vi "运维调试_氨氮.vi"() -> ()   [LabVIEW 2016, in "斯坦道氨氮.lvlib"]
uses:
  <vilib>/Utility/miscctls.llb/LVPointTypeDef.ctl
  <vilib>/Utility/config.llb/NI_LVConfig.lvlib
  <vilib>/ptbypt/NI_PtbyPt.lvlib
panel:
  out "二级权限":bool
  out "一级权限":bool
  out "输入密码":u32
  out "布尔":bool
  in  "仪器参数设置":bool
  in  "流程固件":bool
  in  "量程参数读取":T1
  in  "模块启用":bool
  in  "串口设置":bool
  in  "公式一键写入":bool
  in  "流程路径":path=path "C:/Users/STD/Documents/斯坦道流程文件/流程.xml"
  in  "曲线模型":cluster{"X^2":dbl, "X":dbl, "B":dbl}(xcontrol)
  out "字符串":string
  in  "质控参数设置":bool
  in  "自动测试量程配置":T2
  out "温度2":sgl
  out "温度1":sgl
  out "ADC":sgl
  out "固件版本号":string
  in  "数组":string[](array[string])
  in  "量程切换阈值写入":bool
  in  "量程切换阈值读取":bool
  in  "参数下拉列表":enum16{"总磷", "总氮", "氨氮"}(ring)=enum."氨氮"
  in  "量程下拉列表":enum16{"低量程", "高量程"}(ring)
  in  "测量模式下拉列表":enum16{"水样测量", "零点核查", "跨度核查", "标样核查", "加标回收"}(ring)
  in  "公式":cluster{"X^2":dbl, "X":dbl, "b":dbl}
  in  "写公式":bool
  in  "读公式":bool
  in  "返回":bool
  in  "设置":bool
  out "序列号":string="序列号"
  out "测量数据":T3(xcontrol)
  out "集成报警信息":string
  out "定时启动":bool
  out "总磷总氮运行状态":T4(xcontrol)
  in  "停止":bool
  in  "手动启动":bool
  in  "单步测试":bool
  in  "总磷氨氮调试":u16[](xcontrol)
  out "F3":sgl format="%#.6f"
  out "F2":sgl format="%#.6f"
  out "F1":sgl format="%#.6f"
  out "F0":sgl format="%#.6f"
  out "多列列表框":i32(listbox)
  # "参数设置"
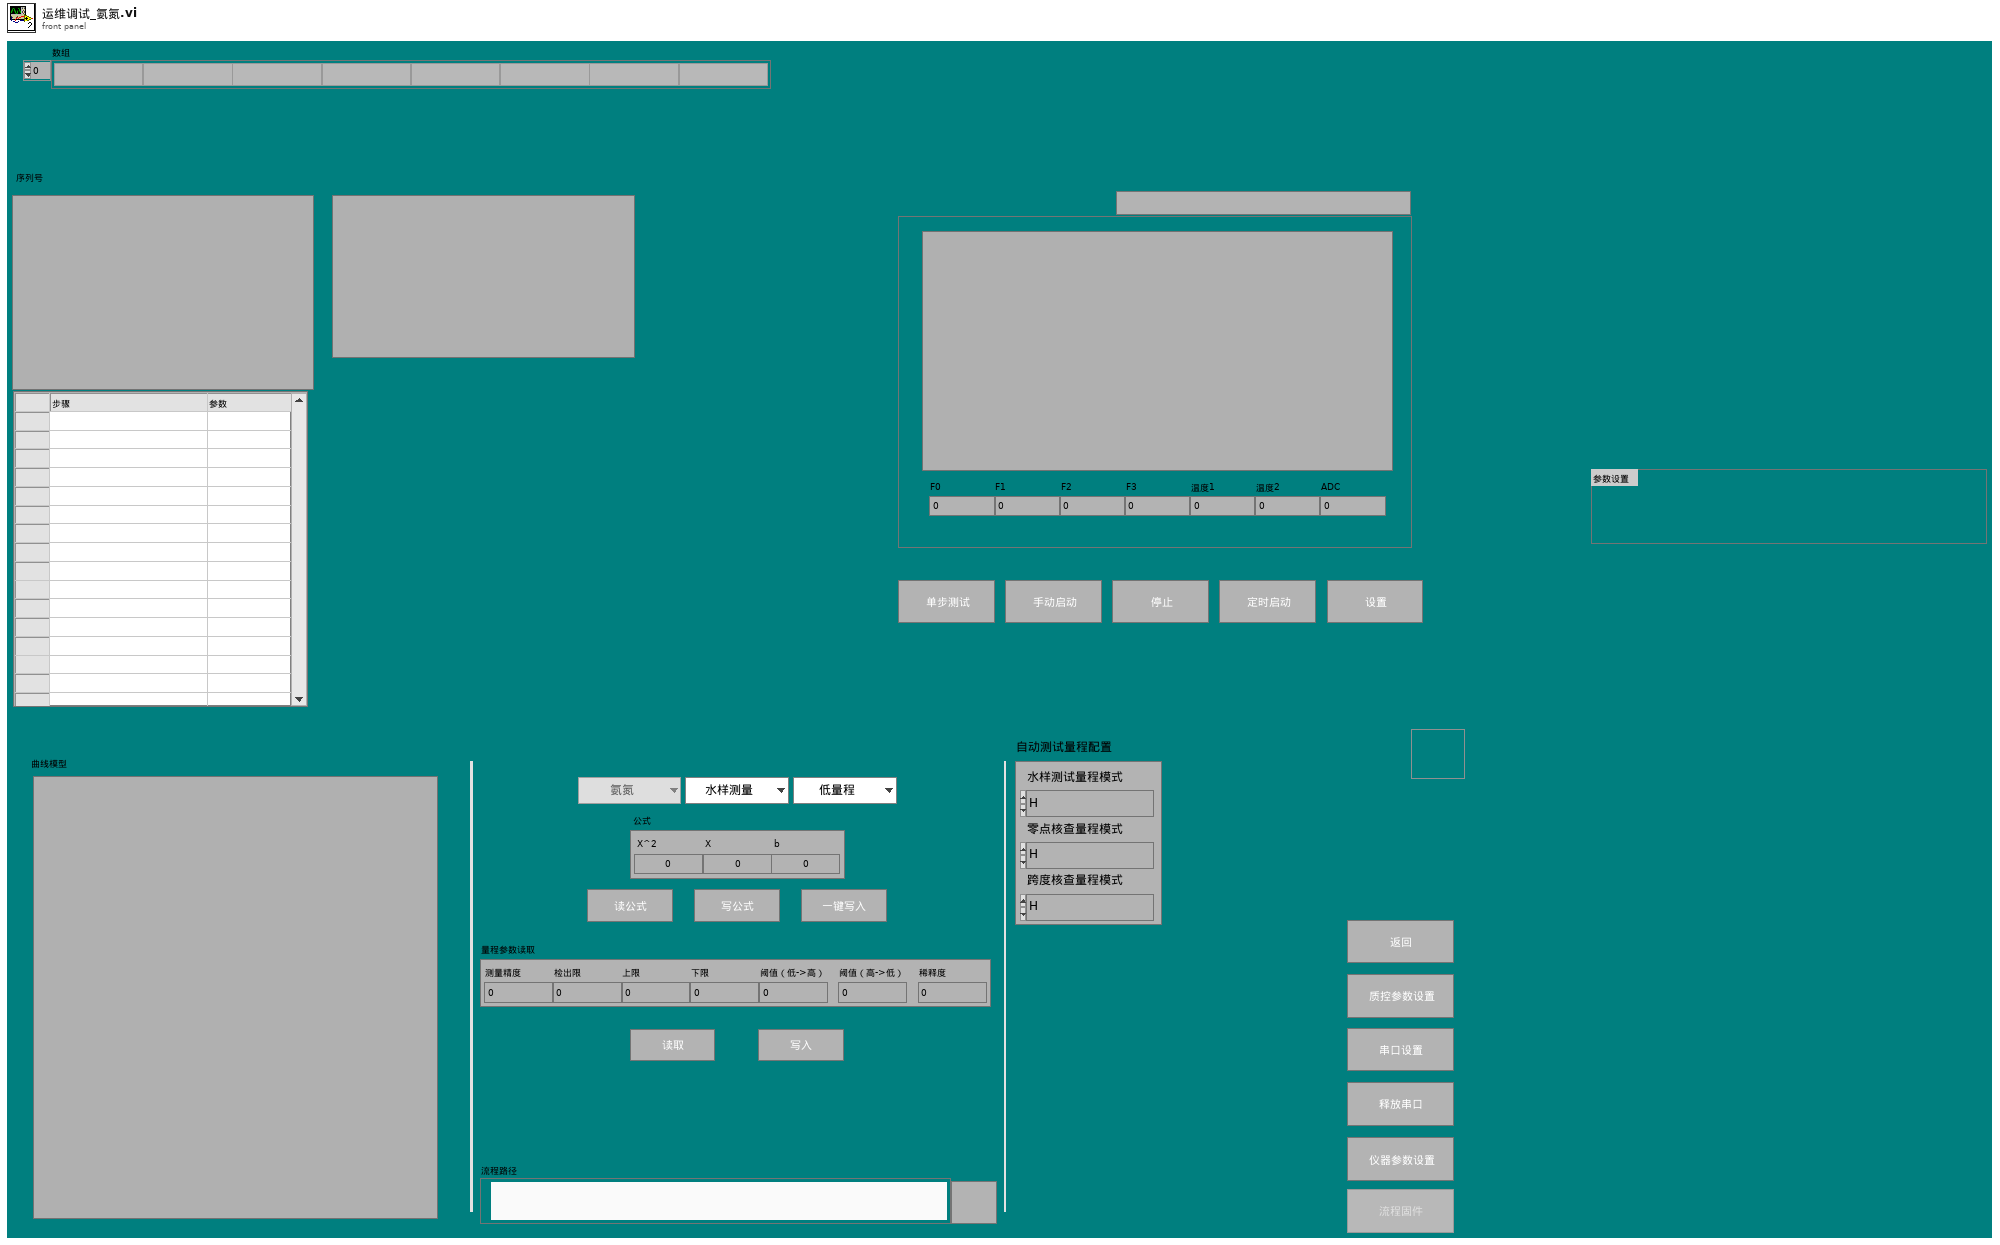
[diagram p1: front panel]
types:
  T1 = cluster{"测量精度":dbl, "检出限":dbl, "上限":dbl, "下限":dbl, "阈值（低->高）":dbl, "阈值（高->低）":dbl, "稀释度":dbl}
  T2 = cluster{"水样测试量程模式":enum16{"H", "L", "AUTO"}, "空白核查量程模式":enum16{"H", "L", "AUTO"}, "跨度核查量程模式":enum16{"H", "L", "AUTO"}}
  T3 = cluster{"flowid":u16, "测量精度":u16, "测量数据区":cluster{"因子编码":u32, "单位":u16, "标样参考值":sgl, "水样数据时间":timestamp, "水样实测值":sgl, "水样数据标识":string, "标样数据时间":timestamp, "标样实测值":sgl, "标样数据标识":string, "空白数据时间":timestamp, "空白实测值":sgl, "空白数据标识":string, "零点核查数据时间":timestamp, "零点核查实测值":sgl, "零点核查数据标识":string, "跨度核查数据时间":timestamp, "跨度核查实测值":sgl, "跨度核查数据标识":string, "加标回收数据时间":timestamp, "加标回收实测值":sgl, "加标回收数据标识":string, "平行样数据时间":timestamp, "平行样实测值":sgl, "平行样数据标识":string, "F0":sgl, "F1":sgl, "F2":sgl, "F3":sgl, "F4":sgl, "F5":sgl, "F6":sgl, "F7":sgl, "温度":sgl, "湿度":sgl, "X值":sgl, "fidrange":sgl}}
  T4 = cluster{"系统时间":timestamp, "工作状态":enum16{"空闲", "水样测试", "标样核查", "零点核查", "跨度核查", "空白测试", "平行样测试", "加标回收", "空白校准", "标样校准", "初始化（清洗）"}, "测量模式":enum16{"待机", "连续模式", "周期模式", "定点模式", "受控模式", "手动模式"}, "告警代码":u16, "故障代码":u16, "日志代码":u16, "软件版本":u16, "F0":sgl, "F1":sgl, "F2":sgl, "F3":sgl, "T":sgl, "H":sgl, "id":u16, "flowid":u16, "量程":u16, "总磷控温温度1":sgl, "营养盐控温温度2":sgl, "ADC":sgl}
  T5 = enum16{"启动测量", "标样核查", "零点核查", "跨度核查", "空白测试", "平行样测试", "加标回收", "空白校准", "标样校准", "初始化（清洗）", "停止测试", "仪器重启", "校时", "模式设置", "测量间隔设置"}
  T6 = cluster{"控制命令":enum16{"启动测量", "标样核查", "零点核查", "跨度核查", "空白测试", "平行样测试", "加标回收", "空白校准", "标样校准", "初始化（清洗）", "停止测试", "仪器重启", "校时", "模式设置", "测量间隔设置"}, "周期设置类型":enum16{"定点启动", "间隔启动"}, "定时功能启用":bool, "定时间隔":dbl, "24H周期设置":bool[], "零点核查时间":u16, "跨度核查时间":u16, "质控频次":enum16{"关闭", "每天", "星期一", "星期二", "星期三", "星期四", "星期五", "星期六", "星期日"}}
  T7 = enum16{"关闭", "每天", "星期一", "星期二", "星期三", "星期四", "星期五", "星期六", "星期日"}
  T8 = typedef "LVDateTimeRec.ctl" = cluster{"秒数的小数部分":dbl, "秒":i32, "分":i32, "时":i32, "日":i32, "月":i32, "年":i32, "天数（周）":i32, "天数（年）":i32, "DST":i32}
  T9 = enum16{"空闲", "水样测试", "标样核查", "零点核查", "跨度核查", "空白测试", "平行样测试", "加标回收", "空白校准", "标样校准", "初始化（清洗）"}
  T10 = enum32{"Bad", "Idle", "Run top level", "Running"}
  T11 = typedef "LVPointTypeDef.ctl" = cluster{"Horizontal":i16, "Vertical":i16}
  T12 = cluster{"因子编码":u32, "单位":u16, "标样参考值":sgl, "水样数据时间":timestamp, "水样实测值":sgl, "水样数据标识":string, "标样数据时间":timestamp, "标样实测值":sgl, "标样数据标识":string, "空白数据时间":timestamp, "空白实测值":sgl, "空白数据标识":string, "零点核查数据时间":timestamp, "零点核查实测值":sgl, "零点核查数据标识":string, "跨度核查数据时间":timestamp, "跨度核查实测值":sgl, "跨度核查数据标识":string, "加标回收数据时间":timestamp, "加标回收实测值":sgl, "加标回收数据标识":string, "平行样数据时间":timestamp, "平行样实测值":sgl, "平行样数据标识":string, "F0":sgl, "F1":sgl, "F2":sgl, "F3":sgl, "F4":sgl, "F5":sgl, "F6":sgl, "F7":sgl, "温度":sgl, "湿度":sgl, "X值":sgl, "fidrange":u16}
  T13 = typedef "NI_LVConfig.lvlib/Config Data RefNum.ctl" = refnum<k1>
  T14 = enum8{"Enabled", "Disabled", "Disabled and Grayed Out"}
  T15 = cluster{"启动模式":enum16{"跨度核查", "水样测量", "空白核查", "标样核查", "加标回收"}, "启动参数":u16, "量程":enum16{"低量程", "高量程"}}
  T16 = cluster{"时间标识":timestamp, "设备":string, "日志信息":string, "流程参数":string}
  T17 = cluster{"时间标识":timestamp, "设备":string, "日志信息":string}
  T18 = typedef "LVRowAndColumnUnsignedTypeDef.ctl" = cluster{"Row":u32, "Column":u32}
  T19 = cluster{"参数下拉列表":enum16{"总磷", "总氮", "氨氮"}, "测量模式下拉列表":enum16{"水样测量", "零点核查", "跨度核查", "标样核查", "加标回收"}, "量程下拉列表":enum16{"低量程", "高量程"}}
  T20 = cluster{"站号":u16, "量程切换":enum32{"H", "L", "AUTO"}, "控制命令":enum16{"启动测量", "标样核查", "零点核查", "跨度核查", "空白测试", "平行样测试", "加标回收", "空白校准", "标样校准", "初始化（清洗）", "停止测试", "仪器重启", "校时", "模式设置", "测量间隔设置"}, "模式设置":enum16{"待机", "连续模式", "周期模式", "定点模式", "受控模式", "手动模式"}, "测量间隔":u16}
  T21 = cluster{"跨度值":dbl, "零点标准液浓度":dbl, "跨度标准液浓度":dbl, "标准液标准浓度":dbl}
  T22 = cluster{"确定":bool, "跨度值":dbl, "零点标准液浓度":dbl, "跨度标准液浓度":dbl, "标准液标准浓度":dbl}
  T23 = cluster{"测量量程":dbl, "测量精度":dbl, "测量间隔":dbl, "消解温度":dbl, "消解时长":dbl, "空白校准时间":timestamp, "曲线截距":dbl, "曲线斜率":dbl, "测量检出限":dbl, "测量信号值":dbl, "线性相关系数":dbl, "二次多项式系数":dbl, "标样校准时间":timestamp, "单位":u16}
  T24 = cluster{"确定":bool, "测量量程":dbl, "测量精度":dbl, "测量间隔":dbl, "消解温度":dbl, "消解时长":dbl, "空白校准时间":timestamp, "曲线截距":dbl, "曲线斜率":dbl, "测量检出限":dbl, "测量信号值":dbl, "线性相关系数":dbl, "二次多项式系数":dbl, "标样校准时间":timestamp, "单位":u16}
  T25 = cluster{"控制命令":enum16{"启动测量", "标样核查", "零点核查", "跨度核查", "空白测试", "平行样测试", "加标回收", "空白校准", "标样校准", "初始化（清洗）", "停止测试", "仪器重启", "校时", "模式设置", "测量间隔设置"}, "周期设置类型":enum16{"定点启动", "间隔启动"}, "定时功能启用":bool, "定时间隔":dbl, "24H周期设置":bool[], "空白核查时间":u16, "跨度核查时间":u16, "质控频次":enum16{"关闭", "每天", "星期一", "星期二", "星期三", "星期四", "星期五", "星期六", "星期日"}}
  T26 = cluster{"测量精度":u16, "检出限":dbl, "上限":dbl, "下限":dbl, "阈值（低->高）":dbl, "阈值（高->低）":dbl, "稀释度":dbl}
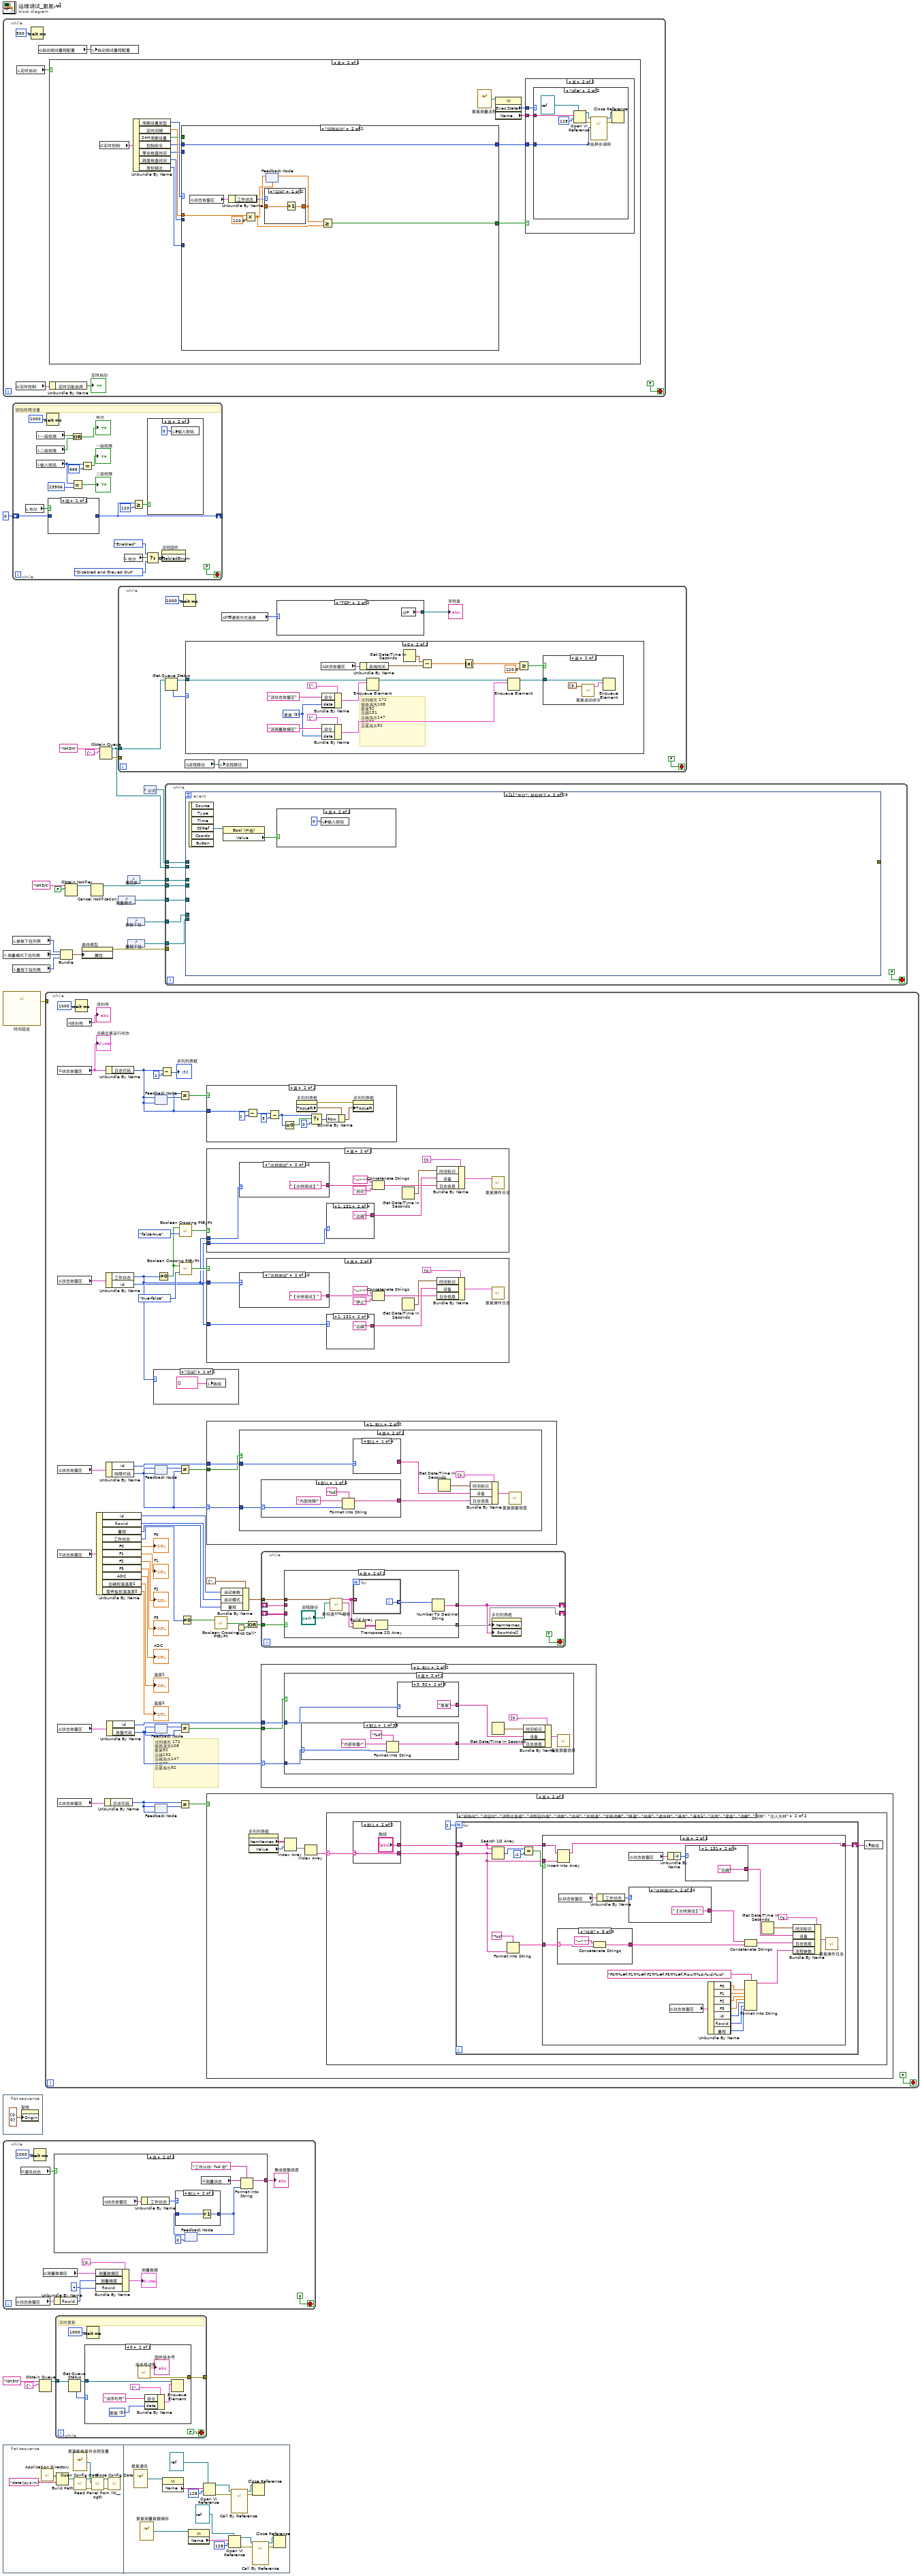
[diagram p0: block diagram]
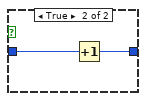
[diagram p3: hidden frame]
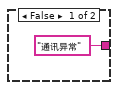
[diagram p5: hidden frame]
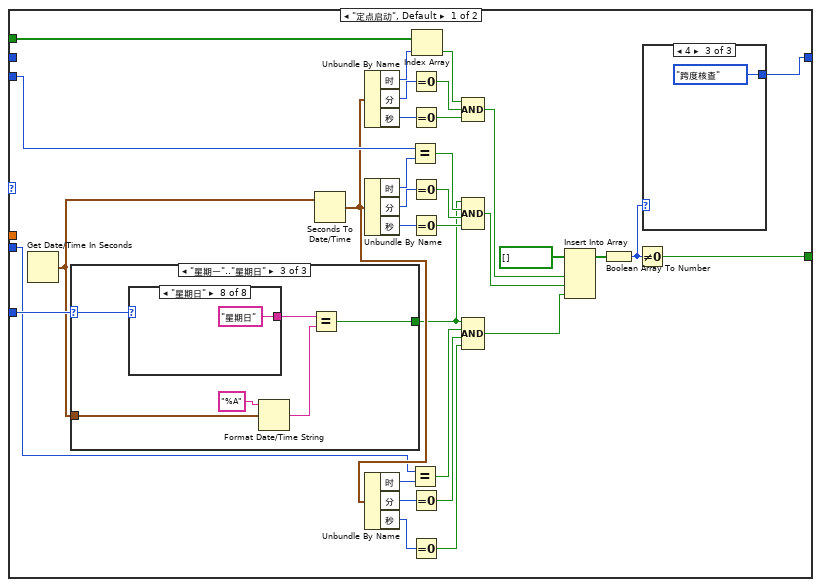
[diagram p8: hidden frame]
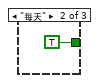
[diagram p10: hidden frame]
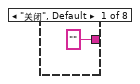
[diagram p11: hidden frame]
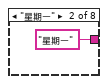
[diagram p12: hidden frame]
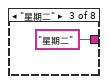
[diagram p13: hidden frame]
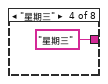
[diagram p14: hidden frame]
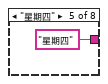
[diagram p15: hidden frame]
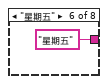
[diagram p16: hidden frame]
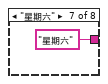
[diagram p17: hidden frame]
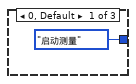
[diagram p18: hidden frame]
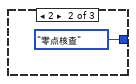
[diagram p19: hidden frame]
diagram:
  n1 = while {
    stop <- FALSE stop-if-true
    n2 = global read "氨氮断电保存全局变量.vi" "定时控制"() -> (w25:T6)
    n3 = local read "定时启动"() -> (w27:bool)
    n4 = Wait (ms)(milliseconds to wait=u32 500 ("等待时间（毫秒）")) -> ()  [unwired: 1 out]
    n5 = global read "氨氮断电保存全局变量.vi" "自动测试量程配置"() -> (w26:T2)
    n6 = case shown="真" w27 {
      frame False {
      }
      frame True {
        n7 = global read "氨氮断电保存全局变量.vi" "定时控制"() -> (w42:T6)
        n8 = Unbundle By Name(w42) -> ("周期设置类型"=w39:enum16{"定点启动", "间隔启动"}, "定时间隔"=w37:dbl, "24H周期设置"=w36:bool[], "控制命令"=w34:T5, "零点核查时间"=w33:u16, "跨度核查时间"=w32:u16, "质控频次"=w31:T7)
        n9 = case shown="\"间隔启动\"" w39 {
          tunnel: w37 -> [_ w100]
          tunnel: w36 -> [w66 _]
          tunnel: [w44 w98] -> w30
          tunnel: w34 -> [_ w96]
          tunnel: [w70 w96] -> w35
          tunnel: w31 -> [w69 _]
          tunnel: w33 -> [w62 _]
          tunnel: w32 -> [w51 _]
          frame "定点启动", Default {
            n10 = Get Date/Time In Seconds() -> (seconds since 1Jan1904=w68:timestamp)
            n11 = case shown="\"星期一\"..\"星期日\"" w69 {
              selector: w69 -> [_ _ w80]
              tunnel: w68 -> [_ _ w81]
              tunnel: [_ TRUE w77] -> w50
              frame "关闭", Default {
              }
              frame "每天" {
              }
              frame "星期一".."星期日" {
                n12 = case shown="\"星期日\"" w80 {
                  tunnel: ["" ("时间格式字符串(%c)") "星期一" ("时间格式字符串(%c)") "星期二" ("时间格式字符串(%c)") "星期三" ("时间格式字符串(%c)") "星期四" ("时间格式字符串(%c)") "星期五" ("时间格式字符串(%c)") "星期六" ("时间格式字符串(%c)") "星期日" ("时间格式字符串(%c)")] -> w79
                  frame "关闭", Default {
                  }
                  frame "星期一" {
                  }
                  frame "星期二" {
                  }
                  frame "星期三" {
                  }
                  frame "星期四" {
                  }
                  frame "星期五" {
                  }
                  frame "星期六" {
                  }
                  frame "星期日" {
                  }
                }
                n13 = Format Date/Time String(time format string (%c)="%A" ("时间格式字符串(%c)"), seconds (now)=w81) -> (date/time string=w78:string)  [unwired: 1 in]
                n14 = Equal?(x=w79, y=w78) -> (x = y?=w77:bool)
              }
            }
            n15 = Seconds To Date/Time(time stamp (now)=w68) -> (date time rec=w52:T8)  [unwired: 1 in]
            n16 = Unbundle By Name(w52) -> ("时"=w75:i32, "分"=w73:i32, "秒"=w74:i32)
            n17 = Unbundle By Name(w52) -> ("时"=w63:i32, "分"=w65:i32, "秒"=w64:i32)
            n18 = Unbundle By Name(w52) -> ("时"=w55:i32, "分"=w53:i32, "秒"=w54:i32)
            n19 = Equal?(x=w62, y=w63) -> (x = y?=w61:bool)
            n20 = Equal?(x=w51, y=w55) -> (x = y?=w56:bool)
            n21 = Equal To 0?(x=w73) -> (x = 0?=w72:bool)
            n22 = Equal To 0?(x=w74) -> (x = 0?=w71:bool)
            n23 = Equal To 0?(x=w65) -> (x = 0?=w60:bool)
            n24 = Equal To 0?(x=w64) -> (x = 0?=w59:bool)
            n25 = Equal To 0?(x=w53) -> (x = 0?=w57:bool)
            n26 = Equal To 0?(x=w54) -> (x = 0?=w58:bool)
            n27 = Index Array(array=w66, index=w75) -> (element=w67:bool)
            n28 = Compound Arithmetic op=AND ("复合运算")(w67, w72, w71) -> (w48:bool)
            n29 = Compound Arithmetic op=AND ("复合运算")(w50, w61, w60, w59) -> (w47:bool)
            n30 = Compound Arithmetic op=AND ("复合运算")(w50, w56, w57, w58) -> (w46:bool)
            n31 = Insert Into Array(array=bool[] [], new element #1=w48, new element #2=w47, new element #3=w46) -> (w45:bool[])  [unwired: 1 in]
            n32 = Boolean Array To Number(Boolean array=w45) -> (number=w43:u32)
            n33 = Not Equal To 0?(x=w43) -> (x != 0?=w44:bool)
            n34 = case shown="4" w43 {
              tunnel: [T5."启动测量" ("控制命令") T5."零点核查" ("控制命令") T5."跨度核查" ("控制命令")] -> w70
              frame 0, Default {
              }
              frame 2 {
              }
              frame 4 {
              }
            }
          }
          frame "间隔启动" {
            n35 = global read "VAR氨氮全局变量.vi" "状态告警区"() -> (w95:T4)
            n36 = Unbundle By Name(w95) -> ("工作状态"=w94:T9)
            n37 = Multiply(x=w100, y=120.0) -> (x*y=w97:dbl)
            n38 = feedback #1(w97) -> (w102:dbl)
            n39 = case shown="\"空闲\"" w94 {
              tunnel: w102 -> [w104 _]
              tunnel: [w103 _] -> w101
              frame "空闲" {
                n40 = Increment(x=w104) -> (x+1=w103:dbl)
              }
              frame "水样测试", Default {
              }
            }
            n41 = feedback-in #1(w101) -> ()
            n42 = Greater Or Equal?(x=w101, y=w97) -> (x >= y?=w98:bool)
          }
        }
        n43 = vi-ref "氨氮测量流程.vi"() -> (w41:refnum<vi>)
        n44 = property class="VI"(reference=w41) -> ("Exec.State"=w38:T10, "Name"=w40:string)  [unwired: 1 in, 2 out]
        n45 = case shown="真" w30 {
          tunnel: w40 -> [_ w107]
          tunnel: w35 -> [_ w106]
          tunnel: w38 -> [_ w105]
          frame False {
          }
          frame True {
            n46 = case shown="\"Idle\"" w105 {
              tunnel: w107 -> [_ w111]
              tunnel: w106 -> [_ w109]
              frame "Bad", Default {
              }
              frame "Idle" {
                n47 = Open VI Reference(type specifier VI Refnum (for type only)=refnum<vi> refnum, vi path=w111, options=128 ("选项")) -> (vi reference=w112:refnum<vi>, error out=w113:errorcluster)  [unwired: 3 in]
                n48 = call-by-ref "开始异步调用"(reference=w112, error in=w113, "控制命令"=w109) -> (reference out=w114:refnum<vi>, error out=w115:errorcluster)  [unwired: 11 in]
                n49 = Close Reference(reference=w114, error in (no error)=w115) -> ()  [unwired: 1 out]
              }
            }
          }
        }
      }
    }
    n50 = Unbundle By Name(w25) -> ("定时功能启用"=→"定时启动":bool)
    n51 = local write "自动测试量程配置"(w26) -> ()
  }
  n52 = local read "测量模式下拉列表"() -> (w3:enum16{"水样测量", "零点核查", "跨度核查", "标样核查", "加标回收"})
  n53 = call "时间延迟"() -> ("error out"=w15:errorcluster)  [unwired: 11 in]
  n54 = flat-sequence {
    frame #0 {
      n55 = property on="窗格" class="Pane"("Origin"=T11 {"Horizontal"=0, "Vertical"=0} ("原点")) -> ()  [unwired: 2 in, 2 out]
    }
  }
  n56 = while {
    stop <- FALSE stop-if-true
    n57 = global read "VAR氨氮全局变量.vi" "状态告警区"() -> (w122:T4)
    n58 = global read "VAR氨氮全局变量.vi" "通讯状态"() -> (w124:bool)
    n59 = Wait (ms)(milliseconds to wait=u32 1000 ("等待时间（毫秒）")) -> ()  [unwired: 1 out]
    n60 = global read "VAR氨氮全局变量.vi" "测量数据区"() -> (w119:T12)
    n61 = case shown="真" w124 {
      tunnel: ["通讯异常" ("集成报警信息") w129] -> w123
      frame False {
      }
      frame True {
        n62 = global read "VAR氨氮全局变量.vi" "状态告警区"() -> (w135:T4)
        n63 = Unbundle By Name(w135) -> ("工作状态"=w134:T9)
        n64 = feedback #2(0) -> (w132:i32)
        n65 = case shown="默认" w134 {
          tunnel: w132 -> [_ w137]
          tunnel: [_ w136] -> w130
          frame "空闲" {
          }
          frame Default {
            n66 = Increment(x=w137) -> (x+1=w136:i32)
          }
        }
        n67 = feedback-in #2(w130) -> ()
        n68 = global read "VAR氨氮全局变量.vi" "测量状态"() -> (w128:string)
        n69 = Format Into String(format string="工作计时: %d 秒" ("格式字符串"), initial string=w128, w130) -> (resulting string=w129:string)  [unwired: 1 in, 1 out]
      }
    }
    "集成报警信息" <- w123
    n70 = Unbundle By Name(w122) -> ("flowid"=w121:u16)
    n71 = Bundle By Name(cluster=T3 {"flowid"=0, "测量精度"=0, "测量数据区"={"因子编码"=0, "单位"=0, "标样参考值"=0.0, "水样数据时间"=timestamp(0 s since 1904-01-01), "水样实测值"=0.0, "水样数据标识"="", "标样数据时间"=timestamp(0 s since 1904-01-01), "标样实测值"=0.0, "标样数据标识"="", "空白数据时间"=timestamp(0 s since 1904-01-01), "空白实测值"=0.0, "空白数据标识"="", "零点核查数据时间"=timestamp(0 s since 1904-01-01), "零点核查实测值"=0.0, "零点核查数据标识"="", "跨度核查数据时间"=timestamp(0 s since 1904-01-01), "跨度核查实测值"=0.0, "跨度核查数据标识"="", "加标回收数据时间"=timestamp(0 s since 1904-01-01), "加标回收实测值"=0.0, "加标回收数据标识"="", "平行样数据时间"=timestamp(0 s since 1904-01-01), "平行样实测值"=0.0, "平行样数据标识"="", "F0"=0.0, "F1"=0.0, "F2"=0.0, "F3"=0.0, "F4"=0.0, "F5"=0.0, "F6"=0.0, "F7"=0.0, "温度"=0.0, "湿度"=0.0, "X值"=0.0, "fidrange"=0.0}} ("测量数据"), "测量数据区"=w119, "测量精度"=u16 4, "flowid"=w121) -> (→"测量数据":T3)
  }
  n72 = flat-sequence {
    frame #0 {
      n73 = call <vilib>:"Application Directory.vi"() -> ("Application Directory"=w145:path)
      n74 = Build Path(base path=w145, name or relative path="data\\sys.ini" ("名称或相对路径")) -> (appended path=w143:path)
      n75 = vi-ref "氨氮断电保存全局变量.vi"() -> (w141:refnum<vi>)
      n76 = call <vilib>:"Open Config Data.vi"("configuration file path"=w143) -> ("error out"=w139:errorcluster, "refnum"=w142:T13)  [unwired: 8 in, 1 out]
      n77 = call <userlib>:"Read Panel from INI__ogtk.vi"("error in (no error)"=w139, "VI ref"=w141, "refnum"=w142) -> ("error out"=w138:errorcluster, "refnum out"=w140:T13)  [unwired: 7 in]
      n78 = call <vilib>:"Close Config Data.vi"("error in (no error)"=w138, "refnum"=w140) -> ()  [unwired: 8 in, 2 out]
    }
    frame #1 {
      n79 = vi-ref "氨氮通讯.vi"() -> (w161:refnum<vi>)
      n80 = vi-ref "氨氮测量数据储存.vi"() -> (w153:refnum<vi>)
      n81 = property class="VI"(reference=w161) -> ("Name"=w160:string)  [unwired: 1 in, 2 out]
      n82 = property class="VI"(reference=w153) -> ("Name"=w146:string)  [unwired: 1 in, 2 out]
      n83 = Open VI Reference(type specifier VI Refnum (for type only)=refnum<vi> refnum, vi path=w160, options=128 ("选项")) -> (vi reference=w158:refnum<vi>, error out=w156:errorcluster)  [unwired: 3 in]
      n84 = Open VI Reference(type specifier VI Refnum (for type only)=refnum<vi> refnum, vi path=w146, options=128 ("选项")) -> (vi reference=w148:refnum<vi>, error out=w150:errorcluster)  [unwired: 3 in]
      n85 = call-by-ref "?"(reference=w158, error in=w156) -> (reference out=w154:refnum<vi>, error out=w155:errorcluster)  [unwired: 12 in]
      n86 = Close Reference(reference=w154, error in (no error)=w155) -> ()  [unwired: 1 out]
      n87 = call-by-ref "?"(reference=w148, error in=w150) -> (reference out=w152:refnum<vi>, error out=w151:errorcluster)  [unwired: 12 in]
      n88 = Close Reference(reference=w152, error in (no error)=w151) -> ()  [unwired: 1 out]
    }
  }
  n89 = while {
    shift-right: [w164] -> _
    shift-left: u32 0 ("等待时间（毫秒）") -> [w165]
    stop <- FALSE stop-if-true
    # "密码权限设置"
    n90 = local read "布尔"() -> (w166:bool)
    n91 = local read "一级权限"() -> (w173:bool)
    n92 = local read "二级权限"() -> (w174:bool)
    n93 = local read "输入密码"() -> (w177:u32)
    n94 = Wait (ms)(milliseconds to wait=u32 1000 ("等待时间（毫秒）")) -> ()  [unwired: 1 out]
    n95 = case shown="假" w166 {
      tunnel: w165 -> [_ w183]
      tunnel: [_ w182] -> w164
      frame False {
      }
      frame True {
        n96 = Increment(x=w183) -> (x+1=w182:u32)
      }
    }
    n97 = Or(x=w173, y=w174) -> (x .or. y?=→"布尔":bool)
    n98 = Equal?(x=w177, y=u32 23506) -> (x = y?=→"二级权限":bool)
    n99 = Equal?(x=w177, y=u32 666) -> (x = y?=→"一级权限":bool)
    n100 = local read "布尔"() -> (w168:bool)
    n101 = Greater Or Equal?(x=w164, y=u32 120) -> (x >= y?=w162:bool)
    n102 = Select(t=T14."Enabled" ("禁用"), s=w168, f=T14."Disabled and Grayed Out") -> (s? t:f=w169:T14)
    n103 = case shown="真" w162 {
      frame False {
      }
      frame True {
        n104 = local write "输入密码"(u32 0 ("输入密码")) -> ()
      }
    }
    n105 = property on="流程固件" class="Bool"("DisabledEnum"=w169) -> ()  [unwired: 2 in, 2 out]
  }
  n106 = local read "参数下拉列表"() -> (w4:enum16{"总磷", "总氮", "氨氮"})
  n107 = local read "量程下拉列表"() -> (w2:enum16{"低量程", "高量程"})
  n108 = Obtain Queue(name (unnamed)="NH3N" ("名称（未命名）"), element data type=cluster{"命令":string, "data":variant} {"命令"="", "data"=variant}) -> (queue out=w12:refnum<queue>)  [unwired: 3 in, 2 out]
  n109 = while {
    tunnel: w15 -> [_]
    stop <- FALSE stop-if-true
    # "试剂填充 172 \n管路清洗108\n氨氮92\n总磷131\n总磷海水147\n总氮76\n总氮海水92"
    n110 = global read "VAR氨氮全局变量.vi" "状态告警区"() -> (w217:T4)
    "总磷总氮运行状态" <- w217
    n111 = global read "VAR氨氮全局变量.vi" "状态告警区"() -> (w204:T4)
    n112 = global read "VAR氨氮全局变量.vi" "状态告警区"() -> (w209:T4)
    n113 = global read "VAR氨氮全局变量.vi" "状态告警区"() -> (w225:T4)
    n114 = global read "VAR氨氮全局变量.vi" "状态告警区"() -> (w214:T4)
    n115 = global read "VAR氨氮全局变量.vi" "状态告警区"() -> (w202:T4)
    n116 = global read "VAR氨氮全局变量.vi" "序列号"() -> (→"序列号":string)
    n117 = Wait (ms)(milliseconds to wait=u32 1000 ("等待时间（毫秒）")) -> ()  [unwired: 1 out]
    n118 = Unbundle By Name(w225) -> ("id"=w222:u16, "flowid"=w224:u16, "量程"=w223:u16, "工作状态"=w192:T9, "F0"=→"F0":sgl, "F1"=→"F1":sgl, "F2"=→"F2":sgl, "F3"=→"F3":sgl, "ADC"=→"ADC":sgl, "总磷控温温度1"=→"温度1":sgl, "营养盐控温温度2"=→"温度2":sgl)
    n119 = Unbundle By Name(w202) -> ("日志代码"=w201:u16)
    n120 = Unbundle By Name(w217) -> ("日志代码"=w198:u16)
    n121 = Unbundle By Name(w204) -> ("工作状态"=w185:T9, "id"=w184:u16)
    n122 = Unbundle By Name(w209) -> ("id"=w208:u16, "故障代码"=w205:u16)
    n123 = Unbundle By Name(w214) -> ("id"=w213:u16, "告警代码"=w210:u16)
    n124 = case shown="\"空闲\"" w185 {
      frame "空闲" {
        n125 = local write "数组"(string[] [] ("数组")) -> ()
      }
      frame "水样测试", Default {
      }
    }
    n126 = feedback-in #3(w198) -> ()
    n127 = feedback #3(w198) -> (w230:u16)
    n128 = feedback #4(w205) -> (w206:u16)
    n129 = feedback-in #4(w205) -> ()
    n130 = feedback #5(w210) -> (w211:u16)
    n131 = feedback-in #5(w210) -> ()
    n132 = feedback #6(w201) -> (w203:u16)
    n133 = feedback-in #6(w201) -> ()
    n134 = Not Equal To 0?(x=w185) -> (x != 0?=w187:bool)
    n135 = Subtract(x=w198, y=1) -> (x-y=→"多列列表框":i32)
    n136 = Not Equal?(x=w198, y=w230) -> (x != y?=w229:bool)
    n137 = Not Equal?(x=w206, y=w205) -> (x != y?=w207:bool)
    n138 = Not Equal?(x=w211, y=w210) -> (x != y?=w212:bool)
    n139 = Not Equal?(x=w201, y=w203) -> (x != y?=w200:bool)
    n140 = call <vilib>:"Boolean Crossing PtByPt.vi"("direction"=enum16{"either", "false-true", "true-false"}."false-true", "input"=w187) -> ("crossing"=w189:bool)  [unwired: 1 in]
    n141 = call <vilib>:"Boolean Crossing PtByPt.vi"("direction"=enum16{"either", "false-true", "true-false"}."true-false", "input"=w187) -> ("crossing"=w186:bool)  [unwired: 1 in]
    n142 = Not Equal To 0?(x=w192) -> (x != 0?=w227:bool)
    n143 = case shown="真" w229 {
      tunnel: w198 -> [_ w440]
      frame False {
      }
      frame True {
        n144 = Subtract(x=w440, y=1) -> (x-y=w438:i32)
        n145 = Subtract(x=w438, y=5) -> (x-y=w442:i32)
        n146 = Greater Or Equal To 0?(x=w442) -> (x >= 0?=w441:bool)
        n147 = property on="多列列表框" class="MCListbox (严格)"() -> (error out=w446:errorcluster, "TopLeft"=w447:T18)  [unwired: 2 in, 1 out]
        n148 = Select(t=w442, s=w441, f=0) -> (s? t:f=w443:i32)
        n149 = Bundle By Name(cluster=w447, "Row"=w443) -> (w448:T18)
        n150 = property on="多列列表框" class="MCListbox (严格)"(error in=w446, "TopLeft"=w448) -> ()  [unwired: 1 in, 2 out]
      }
    }
    n151 = case shown="真" w189 {
      tunnel: w184 -> [_ w260]
      tunnel: w185 -> [_ w259]
      frame False {
      }
      frame True {
        n152 = case shown="\"水样测试\"" w259 {
          tunnel: [_ "【水样测试】" ("字符串") "【标样核查】" ("字符串") "【零点核查】" ("字符串") "【跨度核查】" ("字符串") "【空白测试】" ("字符串") "【平行样测试】" ("字符串") "【加标回收】" ("字符串") "【空白校准】" ("字符串") "【标样校准】" ("字符串")] -> w258
          frame "空闲", Default {
          }
          frame "水样测试" {
          }
          frame "标样核查" {
          }
          frame "零点核查" {
          }
          frame "跨度核查" {
          }
          frame "空白测试" {
          }
          frame "平行样测试" {
          }
          frame "加标回收" {
          }
          frame "空白校准" {
          }
          frame "标样校准" {
          }
        }
        n153 = case shown="1, 131" w260 {
          tunnel: [_ "总磷" ("table输入") "氨氮" ("table输入") "总氮" ("table输入")] -> w262
          frame Default {
          }
          frame 1, 131 {
          }
          frame 3, 92 {
          }
          frame 2, 76 {
          }
        }
        n154 = Concatenate Strings("-->>" ("字符串"), w258, "启动" ("字符串")) -> (w257:string)
        n155 = Get Date/Time In Seconds() -> (seconds since 1Jan1904=w263:timestamp)
        n156 = Bundle By Name(cluster=T16 {"时间标识"=timestamp(0 s since 1904-01-01), "设备"="", "日志信息"="", "流程参数"=""} ("data in"), "时间标识"=w263, "设备"=w262, "日志信息"=w257) -> (w261:T16)
        n157 = call "氨氮操作日志.vi"("data in"=w261) -> ()  [unwired: 11 in]
      }
    }
    n158 = case shown="真" w186 {
      tunnel: w184 -> [_ w238]
      tunnel: w185 -> [_ w237]
      frame False {
      }
      frame True {
        n159 = case shown="\"水样测试\"" w237 {
          tunnel: [_ "【水样测试】" ("字符串") "【标样核查】" ("字符串") "【零点核查】" ("字符串") "【跨度核查】" ("字符串") "【空白测试】" ("字符串") "【平行样测试】" ("字符串") "【加标回收】" ("字符串") "【空白校准】" ("字符串") "【标样校准】" ("字符串")] -> w236
          frame "空闲", Default {
          }
          frame "水样测试" {
          }
          frame "标样核查" {
          }
          frame "零点核查" {
          }
          frame "跨度核查" {
          }
          frame "空白测试" {
          }
          frame "平行样测试" {
          }
          frame "加标回收" {
          }
          frame "空白校准" {
          }
          frame "标样校准" {
          }
        }
        n160 = case shown="1, 131" w238 {
          tunnel: [_ "总磷" ("table输入") "氨氮" ("table输入") "总氮" ("table输入")] -> w240
          frame Default {
          }
          frame 1, 131 {
          }
          frame 3, 92 {
          }
          frame 2, 76 {
          }
        }
        n161 = Concatenate Strings("-->>" ("字符串"), w236, "停止" ("字符串")) -> (w235:string)
        n162 = Get Date/Time In Seconds() -> (seconds since 1Jan1904=w241:timestamp)
        n163 = Bundle By Name(cluster=T16 {"时间标识"=timestamp(0 s since 1904-01-01), "设备"="", "日志信息"="", "流程参数"=""} ("data in"), "时间标识"=w241, "设备"=w240, "日志信息"=w235) -> (w239:T16)
        n164 = call "氨氮操作日志.vi"("data in"=w239) -> ()  [unwired: 11 in]
      }
    }
    n165 = case shown="1, 默认" w205 {
      selector: w205 -> [_ w345]
      tunnel: w208 -> [_ w346]
      tunnel: w207 -> [_ w344]
      frame 0 {
      }
      frame 1, Default {
        n166 = case shown="真" w344 {
          tunnel: w346 -> [_ w353]
          tunnel: w345 -> [_ w348]
          frame False {
          }
          frame True {
            n167 = case shown="默认" w348 {
              selector: w348 -> [w355 _ _ _ _ _]
              tunnel: [w354 "无故障" "电机故障" "温度故障" "通讯故障" "滴定故障"] -> w347
              frame Default {
                n168 = Format Into String(format string="%d" ("格式字符串"), initial string="内部故障-" ("工作状态"), w355) -> (resulting string=w354:string)  [unwired: 1 in, 1 out]
              }
              frame 0 {
              }
              frame 1 {
              }
              frame 2 {
              }
              frame 3 {
              }
              frame 4 {
              }
            }
            n169 = case shown="默认" w353 {
              tunnel: [_ "总磷" ("table输入") "氨氮" ("table输入") "总氮" ("table输入")] -> w349
              frame Default {
              }
              frame 1, 131 {
              }
              frame 3, 92 {
              }
              frame 2, 76 {
              }
            }
            n170 = Get Date/Time In Seconds() -> (seconds since 1Jan1904=w350:timestamp)
            n171 = Bundle By Name(cluster=T17 {"时间标识"=timestamp(0 s since 1904-01-01), "设备"="", "日志信息"=""} ("data in"), "时间标识"=w350, "设备"=w349, "日志信息"=w347) -> (w351:T17)
            n172 = call "氨氮报警信息.vi"("data in"=w351) -> ()  [unwired: 10 in, 1 out]
          }
        }
      }
    }
    n173 = case shown="真" w200 {
      frame False {
      }
      frame True {
        n174 = property on="多列列表框" class="MCListbox (严格)"() -> ("ItemNames"=w280:string[][], "Value"=w281:i32)  [unwired: 2 in, 2 out]
        n175 = Index Array(array=w280, index (row)=w281) -> (element=w279:string[])  [unwired: 1 in]
        n176 = Index Array(array=w279) -> (element=w278:string)  [unwired: 1 in]
        n177 = case shown="\"初始化\", \"读空白\", \"读取比色值\", \"读取空白值\", \"读数\", \"关阀\", \"关恒温\", \"加热消解\", \"降温\", \"结束\", \"进水样\", \"清洗\", \"清洗1\", \"润洗\", \"显色\", \"消解\", \"预热\", \"注入水样\"" w278 {
          selector: w278 -> [_ w284]
          frame Default {
          }
          frame "初始化", "读空白", "读取比色值", "读取空白值", "读数", "关阀", "关恒温", "加热消解", "降温", "结束", "进水样", "清洗", "清洗1", "润洗", "显色", "消解", "预热", "注入水样" {
            n178 = case shown="默认" w284 {
              selector: w284 -> [w288 w290]
              tunnel: [w288 w290] -> w283
              tunnel: [string[] [] ("数组") "数组"] -> w282
              frame "读数" {
              }
              frame Default {
              }
            }
            n179 = for {
              N: 1 -> [_]
              tunnel: w283 -> [w292]
              shift-right: [w291] -> w285
              shift-left: w282 -> [w293]
              n180 = Search 1D Array(1D array=w293, element=w292) -> (index of element=w296:i32)  [unwired: 1 in]
              n181 = Format Into String(format string="%s" ("格式字符串"), w292) -> (resulting string=w297:string)  [unwired: 2 in, 1 out]
              n182 = Equal?(x=w296, y=-1) -> (x = y?=w294:bool)
              n183 = case shown="真" w294 {
                tunnel: w297 -> [_ w305]
                tunnel: w293 -> [w299 w309]
                tunnel: w292 -> [_ w308]
                tunnel: [w299 w307] -> w291
                frame False {
                }
                frame True {
                  n184 = Insert Into Array(array=w309, new element=w308) -> (w307:string[])  [unwired: 1 in]
                  n185 = case shown="\"结束\"" w305 {
                    selector: w305 -> [w334 w337 w340]
                    tunnel: [w334 w336 w339] -> w301
                    frame Default {
                    }
                    frame "初始化" {
                      n186 = Concatenate Strings("-->>" ("字符串"), w337) -> (w336:string)
                    }
                    frame "结束" {
                      n187 = Concatenate Strings("-->>" ("字符串"), w340) -> (w339:string)
                    }
                  }
                  n188 = global read "VAR氨氮全局变量.vi" "状态告警区"() -> (w304:T4)
                  n189 = Unbundle By Name(w304) -> ("工作状态"=w303:T9)
                  n190 = global read "VAR氨氮全局变量.vi" "状态告警区"() -> (w324:T4)
                  n191 = case shown="\"水样测试\"" w303 {
                    tunnel: [_ "【水样测试】" ("字符串") "【标样核查】" ("字符串") "【零点核查】" ("字符串") "【跨度核查】" ("字符串") "【空白测试】" ("字符串") "【平行样测试】" ("字符串") "【加标回收】" ("字符串") "【空白校准】" ("字符串") "【标样校准】" ("字符串")] -> w302
                    frame "空闲", Default {
                    }
                    frame "水样测试" {
                    }
                    frame "标样核查" {
                    }
                    frame "零点核查" {
                    }
                    frame "跨度核查" {
                    }
                    frame "空白测试" {
                    }
                    frame "平行样测试" {
                    }
                    frame "加标回收" {
                    }
                    frame "空白校准" {
                    }
                    frame "标样校准" {
                    }
                  }
                  n192 = Unbundle By Name(w324) -> ("id"=w323:u16)
                  n193 = global read "VAR氨氮全局变量.vi" "状态告警区"() -> (w319:T4)
                  n194 = case shown="1, 131" w323 {
                    tunnel: [_ "总磷" ("table输入") "氨氮" ("table输入") "总氮" ("table输入")] -> w321
                    frame Default {
                    }
                    frame 1, 131 {
                    }
                    frame 3, 92 {
                    }
                    frame 2, 76 {
                    }
                  }
                  n195 = Unbundle By Name(w319) -> ("F0"=w316:sgl, "F1"=w315:sgl, "F2"=w314:sgl, "F3"=w313:sgl, "id"=w312:u16, "flowid"=w311:u16, "量程"=w310:u16)
                  n196 = Concatenate Strings(w302, w301) -> (w300:string)
                  n197 = Format Into String(format string="F0=%#f,F1=%#f,F2=%#f,F3=%#f,Flow=%d-%-d-%-d" ("格式字符串"), w316, w315, w314, w313, w312, w311, w310) -> (resulting string=w317:string)  [unwired: 2 in, 1 out]
                  n198 = Get Date/Time In Seconds() -> (seconds since 1Jan1904=w320:timestamp)
                  n199 = Bundle By Name(cluster=T16 {"时间标识"=timestamp(0 s since 1904-01-01), "设备"="", "日志信息"="", "流程参数"=""} ("data in"), "时间标识"=w320, "设备"=w321, "日志信息"=w300, "流程参数"=w317) -> (w322:T16)
                  n200 = call "氨氮操作日志.vi"("data in"=w322) -> ()  [unwired: 11 in]
                }
              }
            }
            n201 = local write "数组"(w285) -> ()
          }
        }
      }
    }
    n202 = call <vilib>:"Boolean Crossing PtByPt.vi"("input"=w227) -> ("crossing"=w191:bool)  [unwired: 2 in]
    n203 = Bundle By Name(cluster=T15 {"启动模式"=enum."跨度核查", "启动参数"=1, "量程"=enum."低量程"} ("参数簇"), "启动参数"=w222, "启动模式"=w224, "量程"=w223) -> (w216:T15)
    n204 = First Call?() -> (First Call?: T/F=w228:bool)
    n205 = Or(x=w191, y=w228) -> (x .or. y?=w226:bool)
    n206 = while {
      tunnel: w226 -> [w426]
      tunnel: w216 -> [w425]
      shift-right: [w420] -> _
      shift-left: _ -> [w422]
      shift-right: [w421] -> _
      shift-left: _ -> [w423]
      stop <- TRUE stop-if-true
      n207 = case shown="真" w426 {
        tunnel: [w428 w436] -> w421
        tunnel: [w427 w435] -> w420
        tunnel: w425 -> [_ w430]
        tunnel: w423 -> [w428 _]
        tunnel: w422 -> [w427 _]
        frame False {
        }
        frame True {
          n208 = call "斯坦道XML解析.vi"("添加的路径"="流程路径", "参数簇"=w430) -> ("步骤时间"=w431:string[], "步骤名"=w433:string[])  [unwired: 8 in]
          n209 = for {
            tunnel: w433 -> [_] mode=indexing
            tunnel: [w437] -> w434 mode=indexing
            i -> [w437]
          }
          n210 = Build Array(w433, w431) -> (w432:string[][])
          n211 = Transpose 2D Array(2D array=w432) -> (transposed array=w435:string[][])
          n212 = Number To Decimal String(number=w434) -> (decimal integer string=w436:string[])  [unwired: 1 in]
        }
      }
      n213 = property on="多列列表框" class="MCListbox (严格)"("ItemNames"=w420, "RowHdrs[]"=w421) -> ()  [unwired: 2 in, 2 out]
    }
    n214 = case shown="1, 默认" w210 {
      selector: w210 -> [_ w367]
      tunnel: w213 -> [_ w368]
      tunnel: w212 -> [_ w366]
      frame 0 {
      }
      frame 1, Default {
        n215 = case shown="真" w366 {
          tunnel: w368 -> [_ w375]
          tunnel: w367 -> [_ w369]
          frame False {
          }
          frame True {
            n216 = case shown="默认" w369 {
              selector: w369 -> [w377 _ _ _ _ _ _ _ _ _ _ _ _ _ _ _ _ _ _ _ _ _ _ _ _ _ _ _ _ _ _ _ _ _ _ _ _ _]
              tunnel: [w376 "无告警" "缺试剂告警" "缺水样告警" "缺蒸馏水告警" "缺标液告警" "仪表漏液告警" "标定异常告警" "超量程告警" "加热异常" "低试剂预警" "超上限告警" "超下限告警" "仪表内部其他异常" "滴定异常告警" "电极异常告警" "量程切换告警" "参数设置告警" "PH电极电位异常" "电导率电极异常" "浊度光度异常" "溶解氧电极异常" "溶解氧光强异常" "温度异常告警" "PH异常告警" "溶解氧异常告警" "电导率异常告警" "浊度异常告警" "叶绿素异常告警" "藻密度异常告警" "蓝绿藻异常告警" "ORP异常告警" "氨氮异常告警" "清洁刷异常告警" "SD卡异常告警" "蓝牙异常告警" "WiFi异常告警" "流程异常告警"] -> w370
              frame Default {
                n217 = Format Into String(format string="%d" ("格式字符串"), initial string="内部告警-" ("工作状态"), w377) -> (resulting string=w376:string)  [unwired: 1 in, 1 out]
              }
              frame 0 {
              }
              frame 1 {
              }
              frame 2 {
              }
              frame 3 {
              }
              frame 4 {
              }
              frame 5 {
              }
              frame 6 {
              }
              frame 7 {
              }
              frame 8 {
              }
              frame 9 {
              }
              frame 10 {
              }
              frame 11 {
              }
              frame 12 {
              }
              frame 13 {
              }
              frame 14 {
              }
              frame 15 {
              }
              frame 16 {
              }
              frame 17 {
              }
              frame 18 {
              }
              frame 19 {
              }
              frame 20 {
              }
              frame 21 {
              }
              frame 22 {
              }
              frame 23 {
              }
              frame 24 {
              }
              frame 25 {
              }
              frame 26 {
              }
              frame 27 {
              }
              frame 28 {
              }
              frame 29 {
              }
              frame 30 {
              }
              frame 31 {
              }
              frame 32 {
              }
              frame 33 {
              }
              frame 34 {
              }
              frame 35 {
              }
              frame 36 {
              }
            }
            n218 = case shown="3, 92" w375 {
              tunnel: ["总磷" ("table输入") "氨氮" ("table输入") "总氮" ("table输入")] -> w371
              frame 1, 131 {
              }
              frame 3, 92 {
              }
              frame 2, 76, Default {
              }
            }
            n219 = Get Date/Time In Seconds() -> (seconds since 1Jan1904=w372:timestamp)
            n220 = Bundle By Name(cluster=T17 {"时间标识"=timestamp(0 s since 1904-01-01), "设备"="", "日志信息"=""} ("data in"), "时间标识"=w372, "设备"=w371, "日志信息"=w370) -> (w373:T17)
            n221 = call "氨氮报警信息.vi"("data in"=w373) -> ()  [unwired: 10 in, 1 out]
          }
        }
      }
    }
  }
  n222 = while {
    tunnel: w12 -> [w453]
    tunnel: [w451] -> _
    stop <- FALSE stop-if-true
    # "定时更新"
    n223 = Get Queue Status(queue=w453) -> (queue out=w450:refnum<queue>, # elements in queue=w449:i32)  [unwired: 2 in, 6 out]
    n224 = case shown="0" w449 {
      tunnel: [_ w456] -> w451
      tunnel: w450 -> [_ w455]
      frame Default {
      }
      frame 0 {
        w459 = u16 3 items=["总磷"=1, "氨氮"=3] ("站号")
        n225 = call "版本号读取.vi"() -> ("error out"=w456:errorcluster, "固件版本号"=→"固件版本号":string)  [unwired: 10 in]
        n226 = Bundle By Name(cluster=cluster{"命令":string, "data":variant} {"命令"="", "data"=variant} ("元素"), "命令"="读序列号", "data"=w459) -> (w458:cluster{"命令":string, "data":variant})
        n227 = Enqueue Element(queue=w455, element=w458) -> ()  [unwired: 2 in, 3 out]
      }
    }
    n228 = Wait (ms)(milliseconds to wait=u32 1000 ("等待时间（毫秒）")) -> ()  [unwired: 1 out]
  }
  n229 = Bundle("参数下拉列表"=w4, "测量模式下拉列表"=w3, "量程下拉列表"=w2) -> (w5:T19)  [unwired: 1 in]
  n230 = Obtain Notifier(name (unnamed)="NH3N" ("名称（未命名）"), notification data type=FALSE) -> (notifier out=w8:refnum<notifier>)  [unwired: 2 in, 2 out]
  n231 = property on="曲线模型" class="曲线模型 (严格)"("属性"=w5) -> (error out=w11:errorcluster)  [unwired: 2 in, 1 out]
  n232 = Cancel Notification(0:w8) -> (8:w7:refnum<notifier>)  [unwired: 1 in, 2 out]
  n233 = Obtain Queue(name (unnamed)="NH3N" ("名称（未命名）"), element data type=cluster{"命令":string, "data":variant} {"命令"="", "data"=variant}) -> (queue out=w20:refnum<queue>, error out=w21:errorcluster)  [unwired: 3 in, 1 out]
  n234 = while {
    tunnel: w20 -> [w467]
    tunnel: w21 -> [_]
    stop <- FALSE stop-if-true
    n235 = Get Queue Status(queue=w467) -> (queue out=w463:refnum<queue>, # elements in queue=w462:i32)  [unwired: 2 in, 6 out]
    n236 = Wait (ms)(milliseconds to wait=u32 1000 ("等待时间（毫秒）")) -> ()  [unwired: 1 out]
    n237 = global read "氨氮断电保存全局变量.vi" "流程路径"() -> (w466:path)
    n238 = case shown="0" w462 {
      tunnel: w463 -> [_ w470]
      frame Default {
      }
      frame 0 {
        w479 = u16 3 items=["总磷"=1, "氨氮"=3] ("站号")
        # "试剂填充 172 \n管路清洗108\n氨氮92\n总磷131\n总磷海水147\n总氮76\n总氮海水92"
        n239 = global read "VAR氨氮全局变量.vi" "状态告警区"() -> (w471:T4)
        n240 = Bundle By Name(cluster=cluster{"命令":string, "data":variant} {"命令"="", "data"=variant} ("元素"), "命令"="读状态告警区", "data"=w479) -> (w485:cluster{"命令":string, "data":variant})
        n241 = Bundle By Name(cluster=cluster{"命令":string, "data":variant} {"命令"="", "data"=variant} ("元素"), "命令"="读测量数据区", "data"=w479) -> (w482:cluster{"命令":string, "data":variant})
        n242 = Unbundle By Name(w471) -> ("系统时间"=w478:timestamp)
        n243 = Enqueue Element(queue=w470, element=w485) -> (queue out=w480:refnum<queue>)  [unwired: 2 in, 2 out]
        n244 = Get Date/Time In Seconds() -> (seconds since 1Jan1904=w477:timestamp)
        n245 = Subtract(x=w477, y=w478) -> (x-y=w476:dbl)
        n246 = Absolute Value(x=w476) -> (abs(x)=w475:dbl)
        n247 = Enqueue Element(queue=w480, element=w482) -> (queue out=w472:refnum<queue>)  [unwired: 2 in, 2 out]
        n248 = Greater Or Equal?(x=w475, y=120.0) -> (x >= y?=w473:bool)
        n249 = case shown="真" w473 {
          tunnel: w472 -> [_ w488]
          frame False {
          }
          frame True {
            n250 = call "氨氮启动命令.vi"("参数"=T20 {"站号"=3, "量程切换"=enum."AUTO", "控制命令"=enum."校时", "模式设置"=enum."待机", "测量间隔"=0}) -> ("启动命令"=w487:cluster{"命令":string, "data":variant})  [unwired: 10 in]
            n251 = Enqueue Element(queue=w488, element=w487) -> ()  [unwired: 2 in, 3 out]
          }
        }
      }
    }
    n252 = local write "流程路径"(w466) -> ()
    n253 = global read "氨氮断电保存全局变量.vi" "MB通信方式选择"() -> (w464:enum16{"串口", "TCP"})
    n254 = case shown="\"TCP\"" w464 {
      tunnel: [w490 w491] -> w465
      frame "串口", Default {
        n255 = global read "氨氮断电保存全局变量.vi" "VISA Resource"() -> (w490:refnum<visa-resource-name>)
      }
      frame "TCP" {
        n256 = global read "氨氮断电保存全局变量.vi" "IP"() -> (w491:string)
      }
    }
    "字符串" <- w465
  }
  n257 = control-ref of="测量模式下拉列表"() -> (w17:refnum<vi>)
  n258 = control-ref of="量程参数读取"() -> (w6:refnum<vi>)
  n259 = control-ref of="参数下拉列表"() -> (w18:refnum<vi>)
  n260 = control-ref of="量程下拉列表"() -> (w19:refnum<vi>)
  n261 = control-ref of="公式"() -> (w16:refnum<vi>)
  n262 = while {
    tunnel: w20 -> [w498]
    tunnel: w19 -> [w497]
    tunnel: w18 -> [w496]
    tunnel: w17 -> [w495]
    tunnel: w16 -> [w494]
    tunnel: w6 -> [w493]
    tunnel: w11 -> [_]
    tunnel: w7 -> [w492]
    stop <- FALSE stop-if-true
    n263 = event shown="[1] \"布尔\": 鼠标按下" {
      selector: _ -> [_ _ _ _ _ _ _ _ _ _ _ _ _ _ _ _ _ _ _ _ _ _ _]
      dyn-events: _ -> [_ _ _ _ _ _ _ _ _ _ _ _ _ _ _ _ _ _ _ _ _ _ _]
      timeout: _ -> [_ _ _ _ _ _ _ _ _ _ _ _ _ _ _ _ _ _ _ _ _ _ _]
      tunnel: w498 -> [_ _ _ _ w518 w546 _ _ _ _ _ _ w648 _ w673 w680 _ _ _ _ _ _ _]
      tunnel: w497 -> [_ _ _ _ _ _ _ _ _ _ _ _ _ _ _ _ _ _ _ w696 _ _ _]
      tunnel: w496 -> [_ _ _ _ _ _ _ _ _ _ _ _ _ _ _ _ _ _ _ w694 _ w712 w719]
      tunnel: w495 -> [_ _ _ _ _ _ _ _ _ _ _ _ _ _ _ _ _ _ _ w695 _ _ _]
      tunnel: w494 -> [_ _ _ _ _ _ _ _ _ _ _ _ _ _ _ _ _ _ _ w690 _ _ _]
      tunnel: w493 -> [_ _ _ _ _ _ _ _ _ _ _ _ _ _ _ _ _ _ _ _ _ w710 _]
      tunnel: w492 -> [_ _ _ _ _ _ _ _ _ _ _ _ _ _ _ w675 _ _ _ _ _ _ _]
      tunnel: [_ _ _ w504 _ _ _ _ _ _ _ _ _ _ _ _ _ _ _ _ _ _ _] -> _
      event Timeout {
        n264 = event-data() -> ()  [unwired: 1 in, 3 out]
      }
      event "布尔": Mouse Down {
        n265 = event-data() -> ("CtlRef"=w501:refnum<vi>)  [unwired: 1 in, 5 out]
        n266 = property class="Bool (严格)"(reference=w501) -> ("Value"=w500:bool)  [unwired: 1 in, 2 out]
        n267 = case shown="真" w500 {
          frame False {
            n268 = call "密码键盘.vi"() -> ("NewNumber"=→"输入密码":dbl)  [unwired: 1 in]
          }
          frame True {
            n269 = local write "输入密码"(u32 0 ("输入密码")) -> ()
          }
        }
      }
      event "流程固件": Value Change {
        n270 = event-data() -> ()  [unwired: 1 in, 6 out]
        n271 = call "流程固件设置对话框.vi"() -> ()  [unwired: 12 in]
      }
      event "测量模式下拉列表", "量程下拉列表", "参数下拉列表": Value Change {
        n272 = event-data() -> ()  [unwired: 1 in, 6 out]
        n273 = local read "测量模式下拉列表"() -> (w507:enum16{"水样测量", "零点核查", "跨度核查", "标样核查", "加标回收"})
        n274 = local read "参数下拉列表"() -> (w506:enum16{"总磷", "总氮", "氨氮"})
        n275 = local read "量程下拉列表"() -> (w508:enum16{"低量程", "高量程"})
        n276 = Bundle("参数下拉列表"=w506, "测量模式下拉列表"=w507, "量程下拉列表"=w508) -> (w505:T19)  [unwired: 1 in]
        n277 = property on="曲线模型" class="曲线模型 (严格)"("属性"=w505) -> (error out=w504:errorcluster)  [unwired: 2 in, 1 out]
      }
      event "串口设置": Value Change {
        n278 = event-data() -> ()  [unwired: 1 in, 6 out]
        n279 = global read "氨氮断电保存全局变量.vi" "MB通信方式选择"() -> (w509:enum16{"串口", "TCP"})
        n280 = global read "氨氮断电保存全局变量.vi" "VISA Resource"() -> (w515:refnum<visa-resource-name>)
        n281 = global read "氨氮断电保存全局变量.vi" "PORT"() -> (w513:string)
        n282 = global read "氨氮断电保存全局变量.vi" "IP"() -> (w514:string)
        n283 = call "串口配置.vi"("PORT"=w513, "IP"=w514, "MB通信方式选择"=w509, "请选择串口:"=w515) -> ("PORT 2"=w511:string, "IP 2"=w512:string, "确认 2"=w516:bool, "VISA资源名称 2"=w517:refnum<visa-resource-name>, "MB通信方式选择 2"=w510:enum16{"串口", "TCP"})  [unwired: 3 in]
        n284 = case shown="真" w516 {
          tunnel: w517 -> [_ w523]
          tunnel: w518 -> [_ w522]
          tunnel: w512 -> [_ w521]
          tunnel: w511 -> [_ w520]
          tunnel: w510 -> [_ w519]
          frame False {
          }
          frame True {
            n285 = flat-sequence {
              tunnel: w523 -> [w528]
              tunnel: w522 -> [w529]
              tunnel: w521 -> [w527]
              tunnel: w520 -> [w526]
              tunnel: w519 -> [w525]
              frame #0 {
                n286 = global write "氨氮断电保存全局变量.vi" "IP"(w527) -> ()
                n287 = global write "氨氮断电保存全局变量.vi" "PORT"(w526) -> ()
                n288 = global write "氨氮断电保存全局变量.vi" "VISA Resource"(w528) -> ()
                n289 = global write "氨氮断电保存全局变量.vi" "MB通信方式选择"(w525) -> ()
                n290 = Flush Queue(queue=w529) -> (queue out=w524:refnum<queue>)  [unwired: 1 in, 2 out]
                n291 = Enqueue Element(queue=w524, element=cluster{"命令":string, "data":variant} {"命令"="启用模块", "data"=variant} ("元素")) -> ()  [unwired: 2 in, 3 out]
              }
              frame #1 {
                n292 = call <vilib>:"Application Directory.vi"() -> ("Application Directory"=w544:path)
                n293 = Build Path(base path=w544, name or relative path="data\\sys.ini" ("名称或相对路径")) -> (appended path=w542:path)
                n294 = call <vilib>:"Open Config Data.vi"("configuration file path"=w542) -> ("error out"=w538:errorcluster, "refnum"=w541:T13)  [unwired: 8 in, 1 out]
                n295 = vi-ref "氨氮断电保存全局变量.vi"() -> (w540:refnum<vi>)
                n296 = call <userlib>:"Write Panel to INI__ogtk.vi"("error in (no error)"=w538, "VI ref"=w540, "refnum"=w541) -> ("error out"=w537:errorcluster, "refnum out"=w539:T13)  [unwired: 7 in]
                n297 = call <vilib>:"Close Config Data.vi"("error in (no error)"=w537, "refnum"=w539) -> ("error out"=w532:errorcluster, "file path"=w531:path)  [unwired: 8 in]
                n298 = Open/Create/Replace File(file path (use dialog)=w531, error in=w532) -> (refnum out=w535:refnum<file>, error out=w536:errorcluster)  [unwired: 4 in, 1 out]
                n299 = Flush File(refnum=w535, error in=w536) -> (refnum out=w534:refnum<file>, error out=w533:errorcluster)
                n300 = Close File(refnum=w534, error in=w533) -> ()  [unwired: 2 out]
              }
            }
          }
        }
      }
      event "模块启用": Value Change {
        n301 = event-data() -> ("OldVal"=w547:bool)  [unwired: 1 in, 5 out]
        n302 = Flush Queue(queue=w546) -> (queue out=w545:refnum<queue>)  [unwired: 1 in, 2 out]
        n303 = case shown="假" w547 {
          tunnel: w545 -> [w548 w550]
          frame False {
            n304 = Enqueue Element(queue=w548, element=cluster{"命令":string, "data":variant} {"命令"="停用模块", "data"=variant} ("元素")) -> ()  [unwired: 2 in, 3 out]
          }
          frame True {
            n305 = Enqueue Element(queue=w550, element=cluster{"命令":string, "data":variant} {"命令"="启用模块", "data"=variant} ("元素")) -> ()  [unwired: 2 in, 3 out]
          }
        }
      }
      event "流程路径": Value Change {
        n306 = event-data() -> ()  [unwired: 1 in, 6 out]
        n307 = flat-sequence {
          frame #0 {
            n308 = local read "流程路径"() -> (w552:path)
            n309 = global write "氨氮断电保存全局变量.vi" "流程路径"(w552) -> ()
          }
          frame #1 {
            n310 = call <vilib>:"Application Directory.vi"() -> ("Application Directory"=w566:path)
            n311 = Build Path(base path=w566, name or relative path="data\\sys.ini" ("名称或相对路径")) -> (appended path=w564:path)
            n312 = call <vilib>:"Open Config Data.vi"("configuration file path"=w564) -> ("error out"=w560:errorcluster, "refnum"=w563:T13)  [unwired: 8 in, 1 out]
            n313 = vi-ref "氨氮断电保存全局变量.vi"() -> (w562:refnum<vi>)
            n314 = call <userlib>:"Write Panel to INI__ogtk.vi"("error in (no error)"=w560, "VI ref"=w562, "refnum"=w563) -> ("error out"=w559:errorcluster, "refnum out"=w561:T13)  [unwired: 7 in]
            n315 = call <vilib>:"Close Config Data.vi"("error in (no error)"=w559, "refnum"=w561) -> ("error out"=w554:errorcluster, "file path"=w553:path)  [unwired: 8 in]
            n316 = Open/Create/Replace File(file path (use dialog)=w553, error in=w554) -> (refnum out=w557:refnum<file>, error out=w558:errorcluster)  [unwired: 4 in, 1 out]
            n317 = Flush File(refnum=w557, error in=w558) -> (refnum out=w556:refnum<file>, error out=w555:errorcluster)
            n318 = Close File(refnum=w556, error in=w555) -> ()  [unwired: 2 out]
          }
        }
      }
      event "公式一键写入": Value Change {
        n319 = event-data() -> ()  [unwired: 1 in, 6 out]
        n320 = local read "公式"() -> (w567:cluster{"X^2":dbl, "X":dbl, "b":dbl})
        n321 = call "公式复合写入.vi"("公式"=w567) -> ()  [unwired: 11 in]
      }
      event "曲线模型": Value Change {
        n322 = event-data() -> ()  [unwired: 1 in, 6 out]
        n323 = local write "公式"("曲线模型") -> ()
      }
      event "质控参数设置": Value Change {
        n324 = event-data() -> ()  [unwired: 1 in, 6 out]
        n325 = global read "氨氮断电保存全局变量.vi" "质控参数设置"() -> (w569:T21)
        n326 = call "质控参数设置.vi"("质控参数设置"=w569) -> ("输出簇"=w570:T22)  [unwired: 10 in]
        n327 = Unbundle By Name(w570) -> ("确定"=w571:bool)
        n328 = case shown="真" w571 {
          tunnel: w570 -> [_ w573]
          tunnel: w569 -> [_ w572]
          frame False {
          }
          frame True {
            n329 = flat-sequence {
              tunnel: w573 -> [w580]
              tunnel: w572 -> [w579]
              frame #0 {
                n330 = Unbundle By Name(w580) -> ("跨度值"=w578:dbl, "零点标准液浓度"=w577:dbl, "跨度标准液浓度"=w576:dbl, "标准液标准浓度"=w575:dbl)
                n331 = Bundle By Name(cluster=w579, "跨度值"=w578, "零点标准液浓度"=w577, "跨度标准液浓度"=w576, "标准液标准浓度"=w575) -> (w574:T21)
                n332 = global write "氨氮断电保存全局变量.vi" "质控参数设置"(w574) -> ()
              }
              frame #1 {
                n333 = call <vilib>:"Application Directory.vi"() -> ("Application Directory"=w594:path)
                n334 = Build Path(base path=w594, name or relative path="data\\sys.ini" ("名称或相对路径")) -> (appended path=w592:path)
                n335 = call <vilib>:"Open Config Data.vi"("configuration file path"=w592) -> ("error out"=w588:errorcluster, "refnum"=w591:T13)  [unwired: 8 in, 1 out]
                n336 = vi-ref "氨氮断电保存全局变量.vi"() -> (w590:refnum<vi>)
                n337 = call <userlib>:"Write Panel to INI__ogtk.vi"("error in (no error)"=w588, "VI ref"=w590, "refnum"=w591) -> ("error out"=w587:errorcluster, "refnum out"=w589:T13)  [unwired: 7 in]
                n338 = call <vilib>:"Close Config Data.vi"("error in (no error)"=w587, "refnum"=w589) -> ("error out"=w582:errorcluster, "file path"=w581:path)  [unwired: 8 in]
                n339 = Open/Create/Replace File(file path (use dialog)=w581, error in=w582) -> (refnum out=w585:refnum<file>, error out=w586:errorcluster)  [unwired: 4 in, 1 out]
                n340 = Flush File(refnum=w585, error in=w586) -> (refnum out=w584:refnum<file>, error out=w583:errorcluster)
                n341 = Close File(refnum=w584, error in=w583) -> ()  [unwired: 2 out]
              }
            }
          }
        }
      }
      event "仪器参数设置": Value Change {
        n342 = event-data() -> ()  [unwired: 1 in, 6 out]
        n343 = global read "氨氮断电保存全局变量.vi" "氨氮仪器参数"() -> (w595:T23)
        n344 = call "仪器参数设置.vi"("仪器参数设置"=w595) -> ("仪器参数设置输出"=w596:T24)  [unwired: 10 in]
        n345 = Unbundle By Name(w596) -> ("确定"=w597:bool)
        n346 = case shown="真" w597 {
          tunnel: w596 -> [_ w599]
          tunnel: w595 -> [_ w598]
          frame False {
          }
          frame True {
            n347 = flat-sequence {
              tunnel: w599 -> [w616]
              tunnel: w598 -> [w615]
              frame #0 {
                n348 = Unbundle By Name(w616) -> ("测量量程"=w614:dbl, "测量精度"=w613:dbl, "测量间隔"=w612:dbl, "消解温度"=w611:dbl, "消解时长"=w609:dbl, "空白校准时间"=w608:timestamp, "曲线截距"=w607:dbl, "曲线斜率"=w606:dbl, "测量检出限"=w605:dbl, "测量信号值"=w604:dbl, "线性相关系数"=w603:dbl, "二次多项式系数"=w602:dbl, "标样校准时间"=w601:timestamp, "单位"=w600:u16)
                n349 = Bundle By Name(cluster=w615, "测量量程"=w614, "测量精度"=w613, "测量间隔"=w612, "消解温度"=w611, "消解时长"=w609, "空白校准时间"=w608, "曲线截距"=w607, "曲线斜率"=w606, "测量检出限"=w605, "测量信号值"=w604, "线性相关系数"=w603, "二次多项式系数"=w602, "标样校准时间"=w601, "单位"=w600) -> (w610:T23)
                n350 = global write "氨氮断电保存全局变量.vi" "氨氮仪器参数"(w610) -> ()
              }
              frame #1 {
                n351 = call <vilib>:"Application Directory.vi"() -> ("Application Directory"=w630:path)
                n352 = Build Path(base path=w630, name or relative path="data\\sys.ini" ("名称或相对路径")) -> (appended path=w628:path)
                n353 = call <vilib>:"Open Config Data.vi"("configuration file path"=w628) -> ("error out"=w624:errorcluster, "refnum"=w627:T13)  [unwired: 8 in, 1 out]
                n354 = vi-ref "氨氮断电保存全局变量.vi"() -> (w626:refnum<vi>)
                n355 = call <userlib>:"Write Panel to INI__ogtk.vi"("error in (no error)"=w624, "VI ref"=w626, "refnum"=w627) -> ("error out"=w623:errorcluster, "refnum out"=w625:T13)  [unwired: 7 in]
                n356 = call <vilib>:"Close Config Data.vi"("error in (no error)"=w623, "refnum"=w625) -> ("error out"=w618:errorcluster, "file path"=w617:path)  [unwired: 8 in]
                n357 = Open/Create/Replace File(file path (use dialog)=w617, error in=w618) -> (refnum out=w621:refnum<file>, error out=w622:errorcluster)  [unwired: 4 in, 1 out]
                n358 = Flush File(refnum=w621, error in=w622) -> (refnum out=w620:refnum<file>, error out=w619:errorcluster)
                n359 = Close File(refnum=w620, error in=w619) -> ()  [unwired: 2 out]
              }
            }
          }
        }
      }
      event "自动测试量程配置": Value Change {
        n360 = event-data() -> ()  [unwired: 1 in, 6 out]
        n361 = flat-sequence {
          frame #0 {
            n362 = global write "氨氮断电保存全局变量.vi" "自动测试量程配置"("自动测试量程配置") -> ()
          }
          frame #1 {
            n363 = call <vilib>:"Application Directory.vi"() -> ("Application Directory"=w645:path)
            n364 = Build Path(base path=w645, name or relative path="data\\sys.ini" ("名称或相对路径")) -> (appended path=w643:path)
            n365 = call <vilib>:"Open Config Data.vi"("configuration file path"=w643) -> ("error out"=w639:errorcluster, "refnum"=w642:T13)  [unwired: 8 in, 1 out]
            n366 = vi-ref "氨氮断电保存全局变量.vi"() -> (w641:refnum<vi>)
            n367 = call <userlib>:"Write Panel to INI__ogtk.vi"("error in (no error)"=w639, "VI ref"=w641, "refnum"=w642) -> ("error out"=w638:errorcluster, "refnum out"=w640:T13)  [unwired: 7 in]
            n368 = call <vilib>:"Close Config Data.vi"("error in (no error)"=w638, "refnum"=w640) -> ("error out"=w633:errorcluster, "file path"=w632:path)  [unwired: 8 in]
            n369 = Open/Create/Replace File(file path (use dialog)=w632, error in=w633) -> (refnum out=w636:refnum<file>, error out=w637:errorcluster)  [unwired: 4 in, 1 out]
            n370 = Flush File(refnum=w636, error in=w637) -> (refnum out=w635:refnum<file>, error out=w634:errorcluster)
            n371 = Close File(refnum=w635, error in=w634) -> ()  [unwired: 2 out]
          }
        }
      }
      event "手动启动": Value Change {
        n372 = event-data() -> ()  [unwired: 1 in, 6 out]
        n373 = call "氨氮启动参数对话框.vi"() -> ("确认"=w646:bool, "元素"=w647:cluster{"命令":string, "data":variant})  [unwired: 10 in]
        n374 = case shown="真" w646 {
          tunnel: w648 -> [_ w650]
          tunnel: w647 -> [_ w649]
          frame False {
          }
          frame True {
            n375 = Enqueue Element(queue=w650, element=w649) -> ()  [unwired: 2 in, 3 out]
          }
        }
      }
      event "定时启动": Mouse Down {
        n376 = event-data() -> ()  [unwired: 1 in, 6 out]
        n377 = flat-sequence {
          frame #0 {
            n378 = global read "氨氮断电保存全局变量.vi" "定时控制"() -> (w652:T6)
            n379 = call "周期设置.vi"("定时控制输入"=w652) -> ("定时控制输出"=w651:T25)  [unwired: 10 in]
            n380 = global write "氨氮断电保存全局变量.vi" "定时控制"(w651) -> ()
          }
          frame #1 {
            n381 = call <vilib>:"Application Directory.vi"() -> ("Application Directory"=w666:path)
            n382 = Build Path(base path=w666, name or relative path="data\\sys.ini" ("名称或相对路径")) -> (appended path=w664:path)
            n383 = call <vilib>:"Open Config Data.vi"("configuration file path"=w664) -> ("error out"=w660:errorcluster, "refnum"=w663:T13)  [unwired: 8 in, 1 out]
            n384 = vi-ref "氨氮断电保存全局变量.vi"() -> (w662:refnum<vi>)
            n385 = call <userlib>:"Write Panel to INI__ogtk.vi"("error in (no error)"=w660, "VI ref"=w662, "refnum"=w663) -> ("error out"=w659:errorcluster, "refnum out"=w661:T13)  [unwired: 7 in]
            n386 = call <vilib>:"Close Config Data.vi"("error in (no error)"=w659, "refnum"=w661) -> ("error out"=w654:errorcluster, "file path"=w653:path)  [unwired: 8 in]
            n387 = Open/Create/Replace File(file path (use dialog)=w653, error in=w654) -> (refnum out=w657:refnum<file>, error out=w658:errorcluster)  [unwired: 4 in, 1 out]
            n388 = Flush File(refnum=w657, error in=w658) -> (refnum out=w656:refnum<file>, error out=w655:errorcluster)
            n389 = Close File(refnum=w656, error in=w655) -> ()  [unwired: 2 out]
          }
        }
      }
      event "单步测试": Value Change {
        w668 = u16 1 items=["总磷"=1, "氨氮"=3] ("站号")
        n390 = event-data() -> ()  [unwired: 1 in, 6 out]
        n391 = Bundle("站号"=w668, "总磷氨氮调试"="总磷氨氮调试") -> (w667:cluster{"站号":u16, "总磷氨氮调试":u16[]})  [unwired: 1 in]
        n392 = Bundle By Name(cluster=cluster{"命令":string, "data":variant} {"命令"="", "data"=variant} ("元素"), "命令"="debug", "data"=w667) -> (w670:cluster{"命令":string, "data":variant})
        n393 = Enqueue Element(queue=w673, element=w670) -> ()  [unwired: 2 in, 3 out]
      }
      event "停止": Value Change {
        n394 = event-data() -> ()  [unwired: 1 in, 6 out]
        n395 = Enqueue Element(queue=w680, element=cluster{"命令":string, "data":variant} {"命令"="启动", "data"=variant(cluster{"站号":u16, "控制命令输出":u16[]} {"站号"=1, "控制命令输出"=[2816]})} ("元素")) -> (queue out=w677:refnum<queue>)  [unwired: 2 in, 2 out]
        n396 = Cancel Notification(0:w675) -> (8:w676:refnum<notifier>)  [unwired: 1 in, 2 out]
        n397 = Send Notification(notification=TRUE ("通知"), notifier=w676) -> ()  [unwired: 1 in, 2 out]
        n398 = Enqueue Element(queue=w677, element=cluster{"命令":string, "data":variant} {"命令"="启动", "data"=variant(cluster{"站号":u16, "控制命令输出":u16[]} {"站号"=2, "控制命令输出"=[2816]})} ("元素")) -> ()  [unwired: 2 in, 3 out]
      }
      event "设置": Value Change {
        n399 = event-data() -> ()  [unwired: 1 in, 6 out]
        n400 = property on="窗格" class="Pane"("Origin"=T11 {"Horizontal"=0, "Vertical"=628} ("原点")) -> ()  [unwired: 2 in, 2 out]
      }
      event "返回": Value Change {
        n401 = event-data() -> ()  [unwired: 1 in, 6 out]
        n402 = property on="窗格" class="Pane"("Origin"=T11 {"Horizontal"=0, "Vertical"=0} ("原点")) -> ()  [unwired: 2 in, 2 out]
      }
      event "公式.X^2", "公式.X", "公式.b": Mouse Down {
        n403 = event-data() -> ("CtlRef"=w686:refnum<vi>)  [unwired: 1 in, 5 out]
        n404 = property class="DigNum (严格)"(reference=w686) -> (reference out=w684:refnum<vi>, "Value"=w685:dbl)  [unwired: 1 in, 1 out]
        n405 = call "数字键盘.vi"("OldNumber"=w685) -> ("NewNumber"=w683:dbl)
        n406 = property class="DigNum (严格)"(reference=w684, "Val(Sgnl)"=w683) -> ()  [unwired: 1 in, 2 out]
      }
      event "读公式": Value Change {
        n407 = event-data() -> ()  [unwired: 1 in, 6 out]
        n408 = property class="Enum (严格)"(reference=w695) -> ("Value"=w692:enum16{"水样测量", "零点核查", "跨度核查", "标样核查", "加标回收"})  [unwired: 1 in, 2 out]
        n409 = property class="Enum (严格)"(reference=w694) -> ("Value"=w693:enum16{"总磷", "总氮", "氨氮"})  [unwired: 1 in, 2 out]
        n410 = property class="Enum (严格)"(reference=w696) -> ("Value"=w691:enum16{"低量程", "高量程"})  [unwired: 1 in, 2 out]
        n411 = call "公式读取.vi"("量程"=w691, "测量模式"=w692, "测量参数"=w693) -> ("error out"=w688:errorcluster, "公式"=w689:cluster{"X^2":dbl, "X":dbl, "b":dbl})  [unwired: 7 in]
        n412 = property class="Clust (严格)"(reference=w690, "Value"=w689) -> ()  [unwired: 1 in, 2 out]
        n413 = case shown="错误" w688 {
          tunnel: ["读取成功" ("消息") "读取失败" ("消息")] -> w687
          frame No Error {
          }
          frame Error {
          }
        }
        n414 = One Button Dialog(message=w687) -> ()  [unwired: 1 in, 1 out]
      }
      event "写公式": Value Change {
        n415 = event-data() -> ()  [unwired: 1 in, 6 out]
        n416 = call "公式写入.vi"("公式"="公式", "量程"="量程下拉列表", "测量模式"="测量模式下拉列表", "测量参数"="参数下拉列表") -> ("error out"=w701:errorcluster)  [unwired: 7 in]
        n417 = case shown="无错误" w701 {
          tunnel: ["写入成功" ("消息") "写入失败" ("消息")] -> w702
          frame No Error {
          }
          frame Error {
          }
        }
        n418 = One Button Dialog(message=w702) -> ()  [unwired: 1 in, 1 out]
      }
      event "量程切换阈值读取": Value Change {
        n419 = event-data() -> ()  [unwired: 1 in, 6 out]
        n420 = property class="Enum (严格)"(reference=w712) -> ("Value"=w711:enum16{"总磷", "总氮", "氨氮"})  [unwired: 1 in, 2 out]
        n421 = call "量程读取.vi"("测量参数"=w711) -> ("error out"=w707:errorcluster, "量程参数读取"=w709:T26)  [unwired: 9 in]
        n422 = property class="Clust (严格)"(reference=w710, "Value"=w709) -> ()  [unwired: 1 in, 2 out]
        n423 = case shown="错误" w707 {
          tunnel: ["读取成功" ("消息") "读取失败" ("消息")] -> w708
          frame No Error {
          }
          frame Error {
          }
        }
        n424 = One Button Dialog(message=w708) -> ()  [unwired: 1 in, 1 out]
      }
      event "量程切换阈值写入": Value Change {
        n425 = event-data() -> ()  [unwired: 1 in, 6 out]
        n426 = property class="Enum (严格)"(reference=w719) -> ("Value"=w718:enum16{"总磷", "总氮", "氨氮"})  [unwired: 1 in, 2 out]
        n427 = call "量程写入.vi"("量程参数写入"="量程参数读取", "测量参数"=w718) -> ("error out"=w716:errorcluster)  [unwired: 8 in]
        n428 = case shown="无错误" w716 {
          tunnel: ["写入成功" ("消息") "写入失败" ("消息")] -> w717
          frame No Error {
          }
          frame Error {
          }
        }
        n429 = One Button Dialog(message=w717) -> ()  [unwired: 1 in, 1 out]
      }
    }
  }
